vi "MVE Describe TD.vi"(11 "TD":u8[](array[numeric])) -> ()   [LabVIEW 2016]
uses:
  <vilib>/variable/Type Descriptor.ctl
  <vilib>/variable/NI_Variable.lvlib
panel:
  in  "ok":bool caption="确定"
  out "Data Type Image":picture caption="数据类型图像"
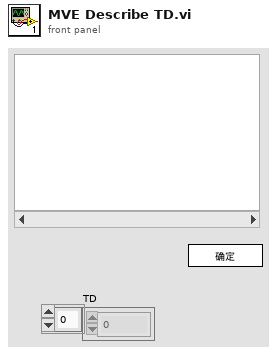
[diagram p1: front panel]
types:
  T1 = typedef "NI_Variable.lvlib/Type Descriptor.ctl" = cluster{"Variant":variant}
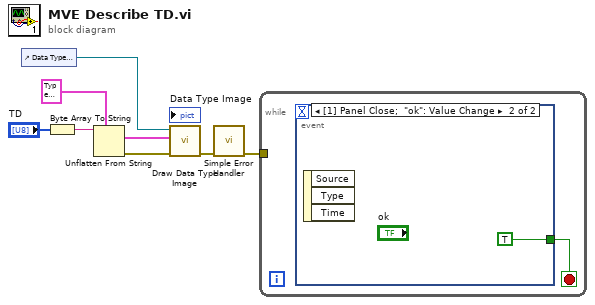
[diagram p0: block diagram]
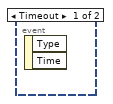
[diagram p2: hidden frame]
diagram:
  n1 = control-ref of="Data Type Image"() -> (w3:refnum<vi>)
  n2 = Byte Array To String(unsigned byte array="TD") -> (string=w7:string)
  n3 = Unflatten From String(type=T1 {"Variant"=variant} ("type descriptor"), binary string=w7) -> (value=w5:T1, error out=w4:errorcluster)  [unwired: 3 in, 1 out]
  n4 = call <vilib>:"Draw Data Type Image.vi"("error in (no error)"=w4, "type descriptor"=w5, "Data Type Image"=w3) -> ("error IO"=w2:errorcluster)  [unwired: 8 in]
  n5 = call <vilib>:"Simple Error Handler.vi"("error in (no error)"=w2) -> ("error out"=w1:errorcluster)  [unwired: 4 in, 4 out]
  n6 = while {
    tunnel: w1 -> [_]
    stop <- w9 stop-if-true
    n7 = event shown="[1] Panel Close;  \"ok\": Value Change" {
      selector: _ -> [_ _]
      dyn-events: _ -> [_ _]
      timeout: _ -> [_ _]
      tunnel: [_ TRUE] -> w9
      event Timeout {
        n8 = event-data() -> ()  [unwired: 1 in, 2 out]
      }
      event Panel Close; "ok": Value Change {
        n9 = event-data() -> ()  [unwired: 1 in, 3 out]
      }
    }
  }
